vi "serial_test.vi"() -> ()   [LabVIEW 2017]
uses:
  Program Files (x86)/National Instruments/LabVIEW 2017/examples/Instrument IO/Serial/support/Serial - Settings.ctl
  <vilib>/Instr/_visa.llb/VISA Configure Serial Port (Instr).vi
panel:
  in  "정지 버튼":bool
  out "숫자":dbl
  out "웨이브폼 그래프":dbl[](graph)
  out "출력 배열":dbl[](array[numeric])
  in  "Serial Settings":T1={"baud rate"=9600, "data bits"=8, "parity"=enum."None", "stop bits"=10, "flow control"=0} {"flow control" items=["None"=0, "XON/XOFF"=1, "RTS/CTS"=2, "DTR/DSR"=4]; "stop bits" items=["1.0"=10, "1.5"=15, "2.0"=20]; "data bits" min=5 max=8 step=1; "baud rate" items=["75"=75, "110"=110, "134"=134, "150"=150, "300"=300, "600"=600, "1200"=1200, "1800"=1800, "2400"=2400, "4800"=4800, "7200"=7200, "9600"=9600, "14400"=14400, "19200"=19200, "28800"=28800, "38400"=38400, "56000"=56000, "57600"=57600, "115200"=115200, "128000"=128000, "230400"=230400]}
  in  "VISA resource name 2":refnum<visa-resource-name>="COM1"
  in  "delay before read (ms)":u32=500
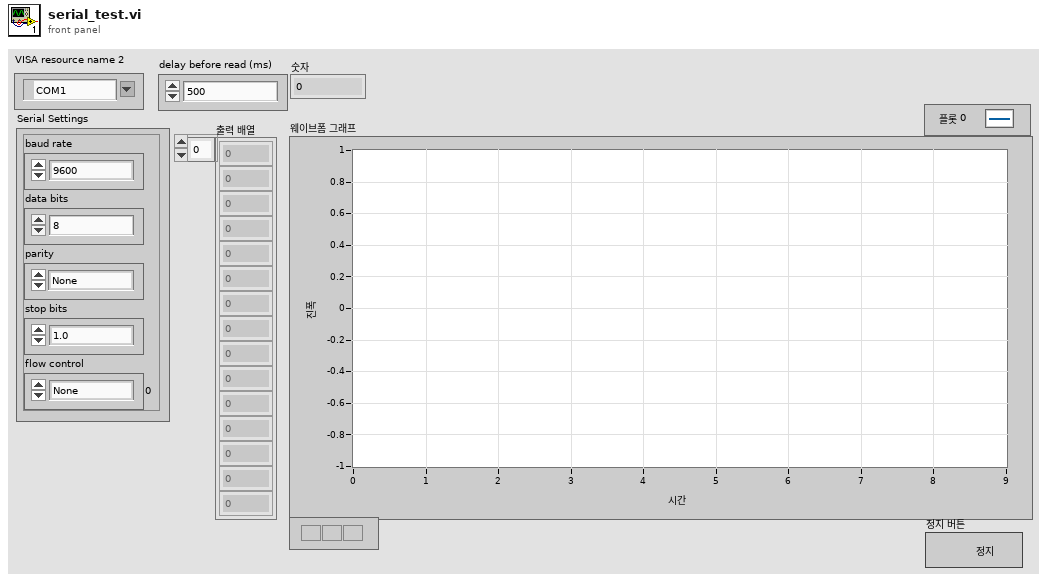
[diagram p1: front panel]
types:
  T1 = typedef "Serial - Settings.ctl" = cluster{"baud rate":u32, "data bits":u16, "parity":enum16{"None", "Odd", "Even", "Mark", "Space"}, "stop bits":u16, "flow control":u16}
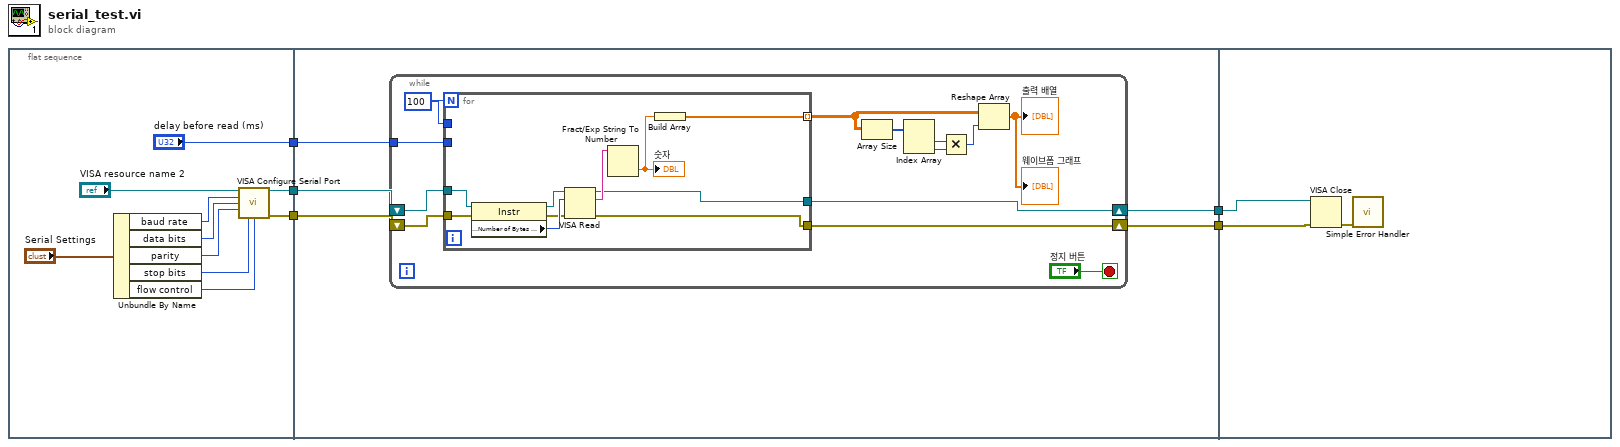
[diagram p0: block diagram]
diagram:
  n1 = flat-sequence {
    tunnel: [w8] -> w5
    tunnel: [w7] -> w4
    tunnel: ["delay before read (ms)"] -> w3
    tunnel: w5 -> [w20]
    tunnel: w4 -> [w19]
    tunnel: w3 -> [w18]
    tunnel: [w17] -> w2
    tunnel: [w16] -> w1
    tunnel: w2 -> [w45]
    tunnel: w1 -> [w44]
    frame #0 {
      n2 = Unbundle By Name("Serial Settings") -> ("baud rate"=w14:u32, "data bits"=w13:u16, "parity"=w12:enum16{"None", "Odd", "Even", "Mark", "Space"}, "stop bits"=w11:u16, "flow control"=w10:u16)
      n3 = call-poly "VISA Configure Serial Port"("VISA resource name"="VISA resource name 2", "baud rate (9600)"=w14, "data bits (8)"=w13, "parity (0:none)"=w12, "stop bits (10: 1 bit)"=w11, "flow control (0:none)"=w10) -> ("VISA resource name out"=w8:refnum<visa-resource-name>, "error out"=w7:errorcluster)  [unwired: 3 in, 5 out]
    }
    frame #1 {
      n4 = while {
        tunnel: w18 -> [w31]
        shift-right: [w22] -> w16
        shift-left: w20 -> [w33]
        shift-right: [w23] -> w17
        shift-left: w19 -> [w32]
        stop <- "정지 버튼" stop-if-true
        w30 = 100
        n5 = for {
          N: w30 -> [_]
          tunnel: w30 -> [_]
          tunnel: w33 -> [w40]
          tunnel: w32 -> [w39]
          tunnel: w31 -> [_]
          tunnel: [w36] -> w25 mode=indexing
          tunnel: [w35] -> w23
          tunnel: [w34] -> w22
          n6 = property class="Instr"(reference=w40, error in=w39) -> (reference out=w41:refnum<visa-resource-name>, error out=w42:errorcluster, "Serial Settings:Number of Bytes at Serial Port"=w43:u32)
          n7 = VISA Read(VISA resource name=w41, byte count=w43, error in (no error)=w42) -> (VISA resource name out=w34:refnum<visa-resource-name>, read buffer=w38:string, error out=w35:errorcluster)  [unwired: 1 out]
          n8 = Fract/Exp String To Number(string=w38) -> (number=w37:dbl)  [unwired: 3 in, 1 out]
          "숫자" <- w37
          n9 = Build Array(w37) -> (w36:dbl[])
        }
        n10 = Array Size(array=w25) -> (size(s)=w28:i32[])
        n11 = Index Array(array=w28) -> (element #1=w27:i32, element #2=w26:i32)  [unwired: 2 in]
        n12 = Multiply(x=w27, y=w26) -> (x*y=w29:i32)
        n13 = Reshape Array(w25, w29) -> (→"웨이브폼 그래프" →"출력 배열":dbl[])
      }
    }
    frame #2 {
      n14 = VISA Close(VISA resource name=w44, error in (no error)=w45) -> (error out=w46:errorcluster)
      n15 = call <vilib>:"Simple Error Handler.vi"("error in (no error)"=w46) -> ()  [unwired: 1 in, 8 out]
    }
  }
